vi "ExEMCircBuf1strip.vi"() -> ()   [LabVIEW 2010]
uses:
  CamHandle.vi
panel:
  out "Waveform Graph":sgl[](graph)
  in  "av gain":dbl format="%.2f"
  in  "Invert Logic output":bool
  in  "Logic Output":i32
  in  "Fan":i32=1
  in  "ADC Gain":u32
  out "ADC Speed (Khz)":u32
  in  "Fast ADC":bool
  in  "Temperature":dbl=-55.0 format="%.2f"
  in  "Exposure":dbl min=0.0 step=0.001 format="%.3f"
  in  "stop":bool
  out "error out":errorcluster
  in  "error in (no error)":errorcluster
  # "ExEMCircBuf1strip:\nThis example allows a center strip\nto be programmed up. It then runs\nin sync (focus) mode displaying \nthe strip data as it comes in.\nNote: this example requires the \ncamera support circular buffers.\nThis example also shows how to \nsetup the cascade to run in over-\nlapped mode and how to set the\non-chip multiplication gain and how\nto set the readout port."
  # "Warning: you must open and run once the VI ExOpenGlobalCam.vi. You only need to run it once then you can run this Example VI as many times as you want."
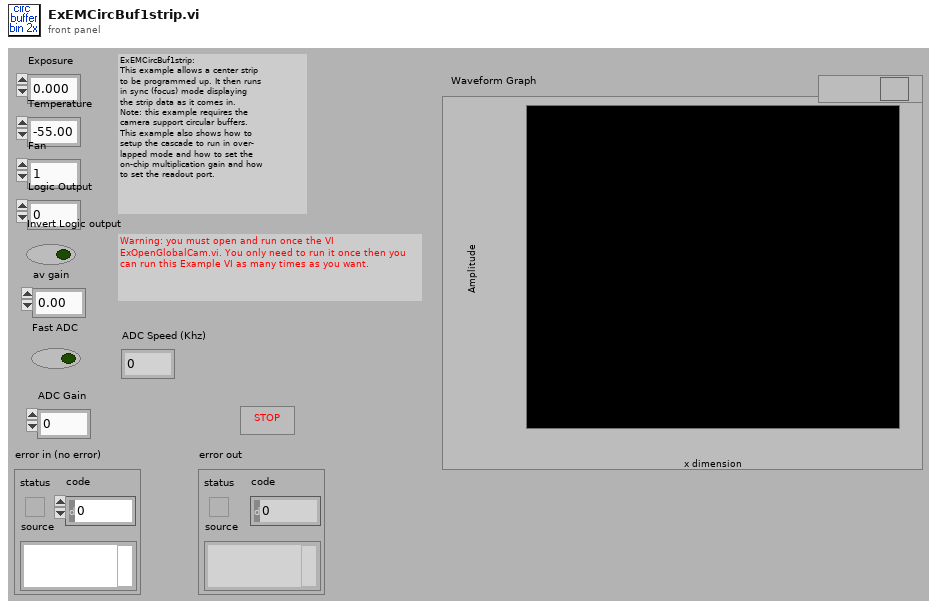
[diagram p1: front panel]
types:
  T1 = cluster{"acquire focus mode":u32, "Exposure":dbl, "Number of Images":u32, "Software accumulation":u32}
  T2 = cluster{"Camera Handle":u32, "Pulser Handle":u32, "File Handle":u32, "Display Handle":u32, "Image Handle":u32}
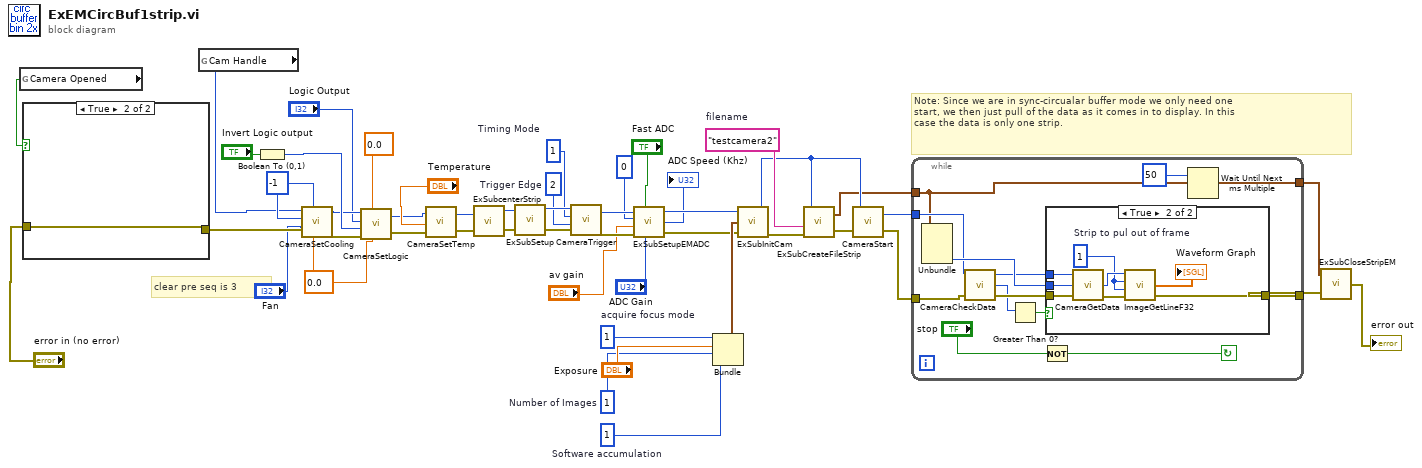
[diagram p0: block diagram]
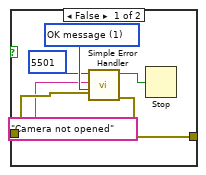
[diagram p3: hidden frame]
diagram:
  w11 = 0.0
  w12 = -1
  w38 = u32 1  # Timing Mode
  w39 = u32 2  # Trigger Edge
  w42 = u32 1  # acquire focus mode
  w41 = u32 1  # Number of Images
  w40 = u32 1  # Software accumulation
  w48 = "testcamera2"  # filename
  # "Note: Since we are in sync-circualar buffer mode we only need one\nstart, we then just pull of the data as it comes in to display. In this \ncase the data is only one strip."
  # "clear pre seq is 3"
  n1 = global read "CamHandle.vi" "Camera Opened"() -> (w21:bool)
  n2 = case shown="True" w21 {
    tunnel: "error in (no error)" -> [w53 w55]
    tunnel: [w52 w55] -> w19
    frame False {
      w54 = u16 1 items=["no dialog", "OK message", "continue or stop message"] ("type of dialog (OK msg:1)")
      n3 = call <vilib>:"Simple Error Handler.vi"("error code (no error:0)"=5501, "error source (\" \")"="Camera not opened", "type of dialog (OK msg:1)"=w54, "error in (no error)"=w53) -> ("error?"=w50:bool, "error out"=w52:errorcluster)  [unwired: 1 in, 3 out]
      n4 = Stop(stop? (T)=w50) -> ()
    }
    frame True {
    }
  }
  n5 = global read "CamHandle.vi" "Cam Handle"() -> (w7:u32)
  n6 = Boolean To (0,1)(Boolean="Invert Logic output") -> (0, 1=w15:i16)
  n7 = call <userlib>:"CameraSetCooling.vi"("Reserved"=w11, "Cooling Mode"=w12, "error in (no error)"=w19, "Fan"="Fan", "Cooling"=w12, "Camera Handle"=w7) -> ("error out"=w18:errorcluster, "Camera Handle"=w14:u32)
  n8 = call <userlib>:"CameraSetLogic.vi"("Reserved 2"=w11, "Reserved"=0.0, "error in (no error)"=w18, "Invert Logic"=w15, "Logic Output"="Logic Output", "Camera Handle"=w14) -> ("error out"=w17:errorcluster, "Camera Handle"=w10:u32)
  n9 = call <userlib>:"CameraSetTemp.vi"("error in (no error)"=w17, "Temperature"="Temperature", "Camera Handle"=w10) -> ("error out"=w35:errorcluster, "Camera Handle"=w34:u32)
  n10 = call "ExSubcenterStrip.vi"("error in (no error)"=w35, "Camera Handle"=w34) -> ("error out"=w32:errorcluster, "Camera Handle"=w36:u32)
  n11 = call "ExSubSetup.vi"("error in (no error)"=w32, "Camera Handle"=w36) -> ("error out"=w31:errorcluster, "Camera Handle"=w44:u32)
  n12 = call <userlib>:"CameraTrigger.vi"("error in"=w31, "Trigger Edge"=w39, "Timing Mode"=w38, "Camera Handle"=w44) -> ("error out"=w29:errorcluster, "Camera Handle"=w30:u32)
  n13 = call "ExSubSetupEMADC.vi"("Camera Handle"=w30, "Fast ADC"="Fast ADC", "ReadOut Port"=0, "Avalanche Gain\nOnly valid for \nport 0"="av gain", "ADC Gain"="ADC Gain", "error in (no error)"=w29) -> ("Camera Handle"=w27:u32, "ADC Speed (Khz)"=→"ADC Speed (Khz)":u32, "error out"=w28:errorcluster)
  n14 = Bundle("acquire focus mode"=w42, "Exposure"="Exposure", "Number of Images"=w41, "Software accumulation"=w40) -> (w46:T1)  [unwired: 1 in]
  n15 = call "ExSubInitCam.vi"("error in (no error)"=w28, "Camera Information"=w46, "Camera Handle"=w27) -> ("error out"=w45:errorcluster, "Camera Handle"=w37:u32)
  n16 = call "ExSubCreateFileStrip.vi"("error in (no error)"=w45, "File and Display Name"=w48, "Camera Handle"=w37) -> ("error out"=w43:errorcluster, "Handles Out"=w4:T2)  [unwired: 1 in]
  n17 = call <userlib>:"CameraStart.vi"("error in"=w43, "Camera Handle"=w37) -> ("error out"=w2:errorcluster, "Camera Handle"=w3:u32)
  n18 = while {
    tunnel: [w64] -> w6
    tunnel: w4 -> [w56]
    tunnel: w3 -> [w58]
    tunnel: w2 -> [w57]
    tunnel: [w56] -> w1
    stop <- w66 continue-if-true
    n19 = Unbundle(w56) -> ("Image Handle"=w63:u32)  [unwired: 4 out]
    n20 = call <userlib>:"CameraCheckData.vi"("Camera Handle"=w58, "error in"=w57) -> ("Camera Handle"=w62:u32, "Number Of Frames Available"=w60:i32, "error out"=w65:errorcluster)
    n21 = Greater Than 0?(x=w60) -> (x > 0?=w61:bool)
    n22 = Not(x="stop") -> (.not. x?=w66:bool)
    n23 = case shown="True" w61 {
      tunnel: w65 -> [w68 w76]
      tunnel: [w68 w74] -> w64
      tunnel: w63 -> [_ w70]
      tunnel: w62 -> [_ w71]
      frame False {
      }
      frame True {
        w72 = 1  # Strip to pul out of frame
        n24 = call <userlib>:"CameraGetData.vi"("error in"=w76, "Data Handle"=w70, "Camera Handle"=w71) -> ("error out"=w75:errorcluster, "Data Handle"=w73:u32)  [unwired: 1 out]
        n25 = call <userlib>:"ImageGetLineF32.vi"("error in"=w75, "Z Position"=w72, "Y Position"=w72, "Data Handle"=w73) -> ("error out"=w74:errorcluster, "Array F32"=→"Waveform Graph":sgl[])  [unwired: 1 out]
      }
    }
    n26 = Wait Until Next ms Multiple(millisecond multiple=50) -> ()  [unwired: 1 out]
  }
  n27 = call "ExSubCloseStripEM.vi"("error in (no error)"=w6, "Handles In"=w1) -> ("error out"=→"error out":errorcluster)
